vi "SymCompt.vi"() -> ()   [LabVIEW 2014]
uses:
  <vilib>/Analysis/Matrix/Datatypes/ComplexMatrix.ctl
  <vilib>/Analysis/Matrix/Datatypes/RealMatrix.ctl
  <vilib>/Analysis/baseanly.llb/Matrix Type of Inverse Matrix.ctl
  <vilib>/Analysis/baseanly.llb/Complex Inverse Matrix.vi
  <vilib>/Analysis/Matrix/Numeric/Conversions/Array To Matrix - CA.vi
  <vilib>/Analysis/Matrix/Numeric/Multiply/Multiply - CM,CM.vi
  <vilib>/Analysis/Matrix/Numeric/Complex/Complex To Polar - CM.vi
  <vilib>/Analysis/NI_AALBase.lvlib
  <vilib>/Analysis/Matrix/NI_Matrix.lvlib
  <vilib>/measure/NI_MABase.lvlib
panel:
  out "theta":dbl[](array[numeric])
  out "r":dbl[](array[numeric])
  out "x/y":cdb[](array[numeric])
  in  "ME %":dbl[](array[numeric])=[0.051, 0.0576, 0.0502]
  in  "PE %":dbl[](array[numeric])=[0.01282, 0.01308, 0.0123]
  in  "E":dbl[][](array[numeric])=[[70.0, 0.0], [70.0, 240.0], [70.0, 0.57]]
  out "Ea Angle (rad)":T1=[[-0.5186245872301148], [-0.5235705683421652], [1.5757707182182803]] format="%.4f"
  out "Ea Mag":T1=[[40.29795494854296], [40.6466580344062], [40.29796912141704]] format="%.4f"
  out "E Matrix":T2=[[70.0+0.0i], [-35.00000000000003-60.62177826491069i], [69.99653607157984+0.6963748846862051i]] format="%.4f"
  out "Ea":T2=[[34.998845357193275-19.975134460074823i], [35.20161168807779-20.322336084410754i], [-0.200457045271067+40.29747054448558i]] format="%.4f"
  out "inv A":T2=[[0.33333333333333337-5.551115123125783e-17i, 0.33333333333333326+0.0i, 0.33333333333333337+5.551115123125783e-17i], [0.33333333333333326+0.0i, -0.16666666666666663+0.28867526918968855i, -0.16666666666666666-0.28867526918968855i], [0.33333333333333337+5.551115123125783e-17i, -0.16666666666666666-0.28867526918968855i, -0.16666666666666669+0.2886752691896885i]] format="%.4f"
  in  "A":T2=[[1.0+0.0i, 1.0+0.0i, 1.0+0.0i], [1.0+0.0i, -0.5-0.866025i, -0.5+0.866025i], [1.0+0.0i, -0.5+0.866025i, -0.5-0.866025i]] format="%.4f"
  # "Phase"
  # "Mag"
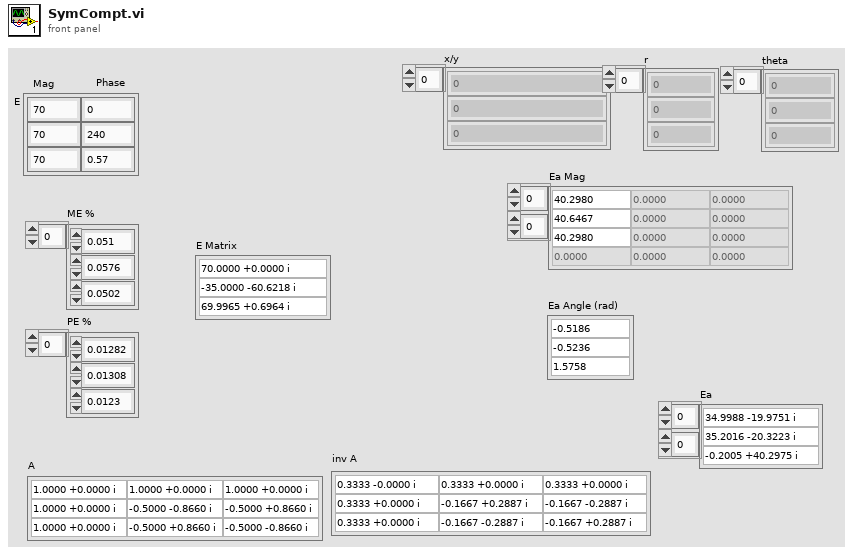
[diagram p1: front panel]
types:
  T1 = typedef "NI_Matrix.lvlib/RealMatrix.ctl" = dbl[][]
  T2 = typedef "NI_Matrix.lvlib/ComplexMatrix.ctl" = cdb[][]
  T3 = typedef "NI_AALBase.lvlib/Matrix Type of Inverse Matrix.ctl" = enum32{"General", "Positive Definite", "Lower Triangular", "Upper Triangular"}
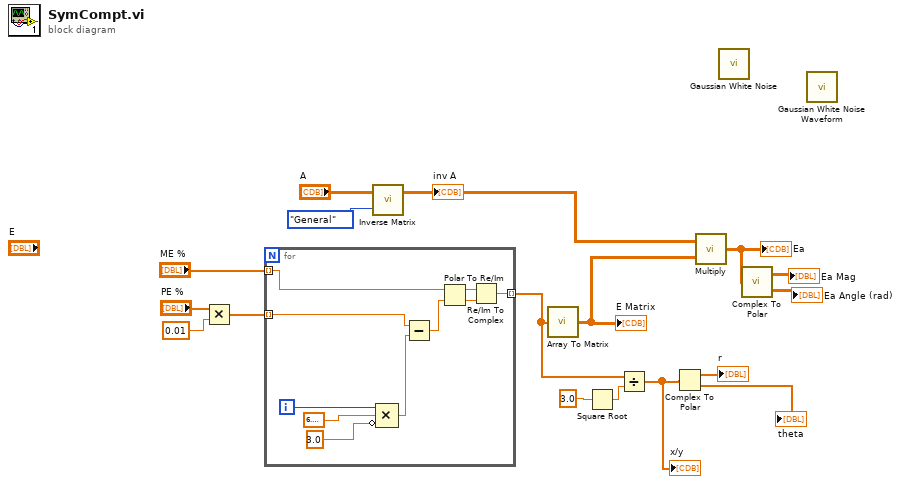
[diagram p0: block diagram]
diagram:
  n1 = Multiply(x="PE %", y=0.01) -> (x*y=w8:dbl[])
  n2 = for {
    tunnel: [w25] -> w4 mode=indexing
    tunnel: "ME %" -> [w24] mode=indexing
    tunnel: w8 -> [w20] mode=indexing
    i -> [w21]
    n3 = Compound Arithmetic op=MULTIPLY(w21, 6.283185307179586, invert 3.0 ("y")) -> (w19:dbl)
    n4 = Subtract(x=w20, y=w19) -> (x-y=w18:dbl)
    n5 = Polar To Re/Im(2:w18, 3:w24) -> (0:w26:dbl, 1:w27:dbl)
    n6 = Re/Im To Complex(1:w26, 2:w27) -> (0:w25:cdb)
  }
  n7 = call-poly <vilib>:"Inverse Matrix.vi"("matrix type"=Matrix_Type_of_Inverse_Matrix."General", "Input Matrix"="A") -> ("Inverse Matrix"=w15:T2)  [unwired: 1 out]
  "inv A" <- w15
  n8 = call-poly <vilib>:"Array To Matrix.vi"("Complex 1D Array"=w4) -> ("Complex Matrix (Column Vector)"=w14:T2)
  "E Matrix" <- w14
  n9 = Square Root(x=3.0) -> (sqrt(x)=w6:dbl)
  n10 = Divide(x=w4, y=w6) -> (x/y=w3:cdb[])
  "x/y" <- w3
  n11 = Complex To Polar(r * e^(i*theta)=w3) -> (r=→"r":dbl[], theta=→"theta":dbl[])
  n12 = call-poly <vilib>:"Multiply.vi"("Complex Matrix B"=w14, "Complex Matrix A"=w15) -> ("A * B"=w13:T2)
  "Ea" <- w13
  n13 = call <vilib>:"Gaussian White Noise.vi"() -> ()  [unwired: 10 in, 2 out]
  n14 = call-poly <vilib>:"Complex To Polar.vi"("Complex Matrix r*e^iQ"=w13) -> ("Modulus r"=→"Ea Mag":T1, "Argument Q"=→"Ea Angle (rad)":T1)
  n15 = call <vilib>:"Gaussian White Noise Waveform.vi"() -> ()  [unwired: 10 in, 2 out]
